vi "Write ShortTestResult.vi"(8 "error in (no error)":errorcluster, 10 "ShortTestReport":string[](array[string]), 11 "TestReport in":refnum<class "TestReport.lvclass">) -> (0 "error out":errorcluster, 3 "TestReport out":refnum<class "TestReport.lvclass">)   [LabVIEW 2019, in "LocalReport.lvlib" / "TestReport.lvclass"]
uses:
  TestReport.lvclass
  TestReport.lvclass/TestReport.ctl
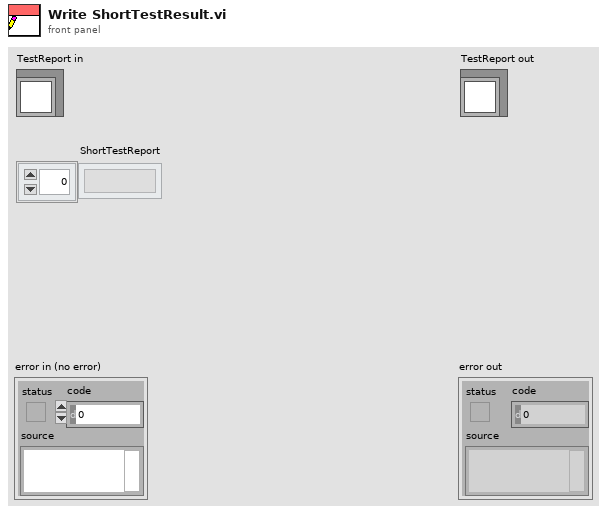
[diagram p1: front panel]
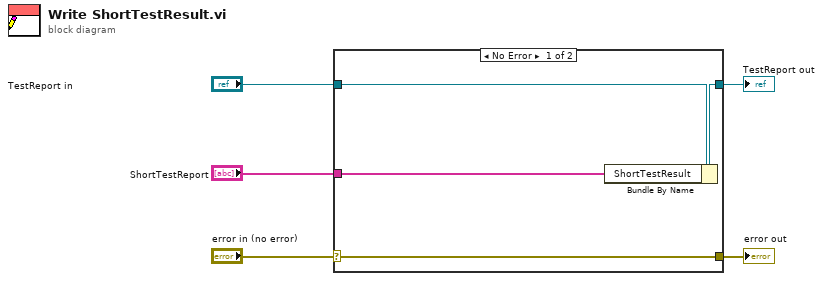
[diagram p0: block diagram]
diagram:
  n1 = case shown="No Error" "error in (no error)" {
    selector: "error in (no error)" -> [w9 w10]
    tunnel: [w9 w10] -> w4
    tunnel: [w7 w11] -> w2
    tunnel: "TestReport in" -> [w8 w11]
    tunnel: "ShortTestReport" -> [w6 _]
    frame No Error {
      n2 = Bundle By Name(cluster=w8, "ShortTestResult"=w6) -> (w7:refnum<class "TestReport.lvclass">)
    }
    frame Error {
    }
  }
  "error out" <- w4
  "TestReport out" <- w2
